vi "CLI Demo.vi"() -> ()   [LabVIEW 2015]
doc: "Demo application for the G-CLI"
uses:
  CLI Class/CLI.lvclass
panel:
  out "StdIn Message":string
  in  "Path":path
  in  "Send File":bool
  in  "Exit Error":errorcluster
  in  "Length (chars)":i32=2048
  in  "Send Random":bool
  out "CLI Input Arguments":string[](array[string])
  in  "stop":bool
  in  "Send Line":bool
  in  "Line":string
  # "To try out the CLI tool. Call this VI from the command line. The exact path depends on your LabVIEW version.\n\nPress Ctrl+I and look under the general tab to get the path."
  # "Writes a single line to the command line."
  # "Writes a large random string to the command line."
  # "Writes the contents of a text file to the command line."
  # "When you stop - the exit error will define the return code."
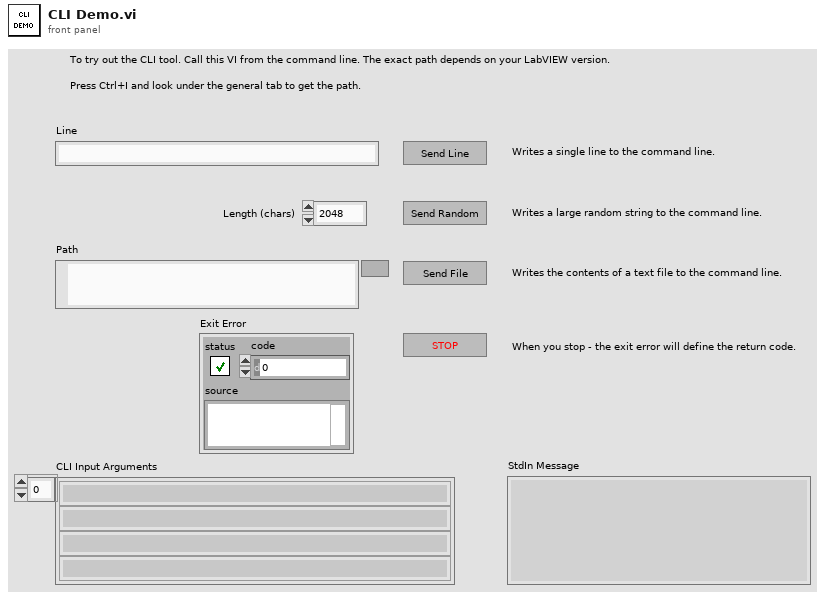
[diagram p1: front panel]
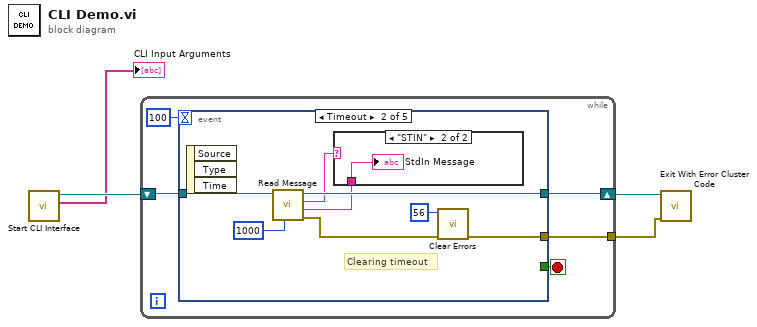
[diagram p0: block diagram]
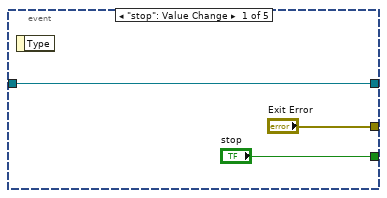
[diagram p2: hidden frame]
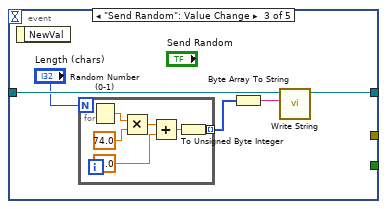
[diagram p4: hidden frame]
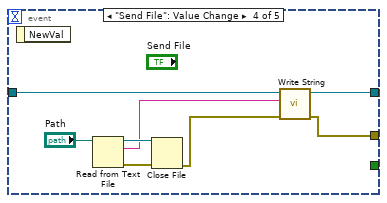
[diagram p5: hidden frame]
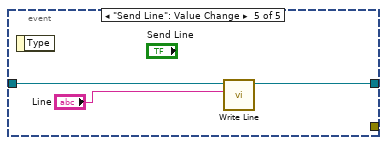
[diagram p6: hidden frame]
diagram:
  n1 = call "Start CLI Interface.vi"() -> ("Custom Parameters"=→"CLI Input Arguments":string[], "CLI out"=w4:refnum<class "CLI.lvclass">)  [unwired: 8 in, 2 out]
  n2 = while {
    shift-right: [w8] -> w3
    shift-left: w4 -> [w7]
    tunnel: [w6] -> w1
    stop <- w9 stop-if-true
    n3 = event shown="[1] Timeout" {
      selector: _ -> [_ _ _ _ _]
      dyn-events: _ -> [_ _ _ _ _]
      timeout: 100 -> [_ _ _ _ _]
      tunnel: ["stop" _ _ _ _] -> w9
      tunnel: [w11 w19 w26 w40 w43] -> w8
      tunnel: w7 -> [w11 w20 w25 w39 w42]
      tunnel: ["Exit Error" w15 _ w34 _] -> w6
      event "stop": Value Change {
        n4 = event-data() -> ()  [unwired: 1 in, 1 out]
      }
      event Timeout {
        # "Clearing timeout"
        n5 = event-data() -> ()  [unwired: 1 in, 3 out]
        n6 = call "Read Message.vi"("timeout ms (25000)"=1000, "CLI in"=w20) -> ("error out"=w18:errorcluster, "Message Contents"=w17:string, "Message Type"=w13:string, "CLI out"=w19:refnum<class "CLI.lvclass">)  [unwired: 6 in]
        n7 = case shown="\"STIN\"" w13 {
          tunnel: w17 -> [_ w21]
          frame "False", Default {
          }
          frame "STIN" {
            "StdIn Message" <- w21
          }
        }
        n8 = call <vilib>:"Clear Errors.vi"("error in (no error)"=w18, "specific error code to clear (0: all)"=56) -> ("error out"=w15:errorcluster)  [unwired: 4 in, 1 out]
      }
      event "Send Random": Value Change {
        n9 = event-data() -> ()  [unwired: 1 in, 1 out]
        n10 = for {
          N: "Length (chars)" -> [_]
          tunnel: [w27] -> w23 mode=indexing
          n11 = Random Number (0-1)() -> (number: 0 to 1=w28:dbl)
          n12 = Multiply(x=w28, y=74.0) -> (x*y=w30:dbl)
          n13 = Add(x=w30, y=48.0) -> (x+y=w32:dbl)
          n14 = To Unsigned Byte Integer(number=w32) -> (unsigned 8bit integer=w27:u8)
        }
        n15 = Byte Array To String(unsigned byte array=w23) -> (string=w22:string)
        n16 = call "Write String.vi"("Text to Write"=w22, "CLI in"=w25) -> ("CLI out"=w26:refnum<class "CLI.lvclass">)  [unwired: 8 in, 1 out]
      }
      event "Send File": Value Change {
        n17 = event-data() -> ()  [unwired: 1 in, 1 out]
        n18 = Read from Text File(file (use dialog)="Path") -> (refnum out=w36:refnum<file>, text=w33:string, error out=w37:errorcluster)  [unwired: 3 in, 1 out]
        n19 = Close File(refnum=w36, error in=w37) -> (error out=w35:errorcluster)  [unwired: 1 out]
        n20 = call "Write String.vi"("error in (no error)"=w35, "Text to Write"=w33, "CLI in"=w39) -> ("error out"=w34:errorcluster, "CLI out"=w40:refnum<class "CLI.lvclass">)  [unwired: 7 in]
      }
      event "Send Line": Value Change {
        n21 = event-data() -> ()  [unwired: 1 in, 1 out]
        n22 = call "Write Line.vi"("Text to Write"="Line", "CLI in"=w42) -> ("CLI out"=w43:refnum<class "CLI.lvclass">)  [unwired: 8 in, 1 out]
      }
    }
  }
  n23 = call "Exit With Error Cluster Code.vi"("error in (no error)"=w1, "CLI in"=w3) -> ()  [unwired: 9 in, 1 out]
